vi "Unlock.vi"(8 "error in (no error)":errorcluster, 10 "New VI Path":path, 11 "Password Protected VI Path":path) -> (0 "error out":errorcluster, 3 "Unlocked VI Path":path)   [LabVIEW 2021, in "VI-Hacker.lvlib"]
doc: "Unlock a password protected VI and save it to a new path."
uses:
  VI-Hacker.lvlib
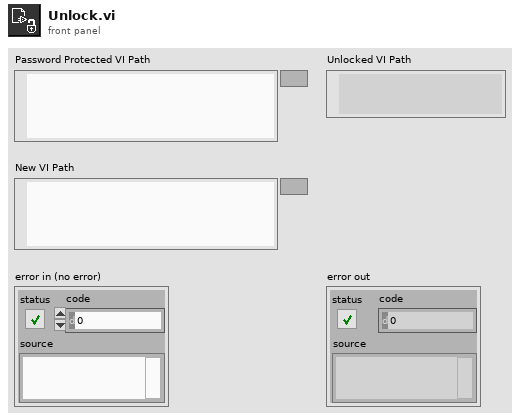
[diagram p1: front panel]
types:
  T1 = typedef "VI-Hacker.lvlib/Content.ctl" = cluster{"Binary Data":string, "Blocks":T2[]}
  T2 = typedef "VI-Hacker.lvlib/Block.ctl" = cluster{"Name":string, "Offset":i32, "Size":i32, "LenSize":i32}
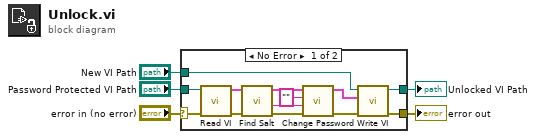
[diagram p0: block diagram]
diagram:
  n1 = case shown="No Error" "error in (no error)" {
    selector: "error in (no error)" -> [w18 w19]
    tunnel: "Password Protected VI Path" -> [w8 _]
    tunnel: [w7 w19] -> w3
    tunnel: "New VI Path" -> [w9 _]
    tunnel: [w10 _] -> w1
    frame No Error {
      n2 = call "Read VI.vi"("error in (no error)"=w18, "VI Path in"=w8) -> ("error out"=w17:errorcluster, "Content out"=w16:T1)  [unwired: 8 in]
      n3 = call "Find Salt.vi"("error in (no error)"=w17, "Content in"=w16) -> ("error out"=w14:errorcluster, "Salt"=w13:string, "Content out"=w15:T1)  [unwired: 6 in, 1 out]
      n4 = call "Change Password.vi"("error in (no error)"=w14, "Salt"=w13, "New Password"="" ("New Password (\"\"=No password)"), "Content in"=w15) -> ("error out"=w12:errorcluster, "Content out"=w11:T1)  [unwired: 6 in]
      n5 = call "Write VI.vi"("error in (no error)"=w12, "Content in"=w11, "VI Path in"=w9) -> ("error out"=w7:errorcluster, "VI Path out"=w10:path)  [unwired: 7 in]
    }
    frame Error {
    }
  }
  "error out" <- w3
  "Unlocked VI Path" <- w1
